vi "GetProbePlanCoordinates.vi"(8 "Use index as X coord":bool=TRUE, 9 "Probe Card Channels":i32=1) -> (0 "file path":string, 2 "OK?":bool, 3 "Array":T1(array[cluster]))   [LabVIEW 2018] (continued)
662\tX=42477.91\ty=10510.80 \nLabel=Strip\t663\tX=42126.23\ty=10577.37 \nLabel=Strip\t664\tX=42473.81\ty=10675.69 \nLabel=Strip\t665\tX=42122.11\ty=10742.12 \nLabel=Strip\t666\tX=42469.65\ty=10840.57 \nLabel=Strip\t667\tX=42117.92\ty=10906.87 \nLabel=Strip\t668\tX=42465.43\ty=11005.45 \nLabel=Strip\t669\tX=42113.68\ty=11071.62 \nLabel=Strip\t670\tX=42461.15\ty=11170.33 \nLabel=Strip\t671\tX=42109.37\ty=11236.36 \nLabel=Strip\t672\tX=42456.80\ty=11335.21 \nLabel=Strip\t673\tX=42104.99\ty=11401.11 \nLabel=Strip\t674\tX=42452.39\ty=11500.10 \nLabel=Strip\t675\tX=42100.55\ty=11565.85 \nLabel=Strip\t676\tX=42447.91\ty=11664.98 \nLabel=Strip\t677\tX=42096.05\ty=11730.60 \nLabel=Strip\t678\tX=42443.37\ty=11829.86 \nLabel=Strip\t679\tX=42091.49\ty=11895.34 \nLabel=Strip\t680\tX=42438.77\ty=11994.74 \nLabel=Strip\t681\tX=42086.86\ty=12060.09 \nLabel=Strip\t682\tX=42434.10\ty=12159.62 \nLabel=Strip\t683\tX=42082.16\ty=12224.83 \nLabel=Strip\t684\tX=42429.37\ty=12324.50 \nLabel=Strip\t685\tX=42077.41\ty=12389.58 \nLabel=Strip\t686\tX=42424.57\ty=12489.37 \nLabel=Strip\t687\tX=42072.59\ty=12554.32 \nLabel=Strip\t688\tX=42419.71\ty=12654.25 \nLabel=Strip\t689\tX=42067.70\ty=12719.06 \nLabel=Strip\t690\tX=42414.79\ty=12819.13 \nLabel=Strip\t691\tX=42062.75\ty=12883.80 \nLabel=Strip\t692\tX=42409.80\ty=12984.01 \nLabel=Strip\t693\tX=42057.74\ty=13048.55 \nLabel=Strip\t694\tX=42404.75\ty=13148.88 \nLabel=Strip\t695\tX=42052.67\ty=13213.29 \nLabel=Strip\t696\tX=42399.64\ty=13313.76 \nLabel=Strip\t697\tX=42047.53\ty=13378.03 \nLabel=Strip\t698\tX=42394.46\ty=13478.63 \nLabel=Strip\t699\tX=42042.33\ty=13542.77 \nLabel=Strip\t700\tX=42389.22\ty=13643.51 \nLabel=Strip\t701\tX=42037.06\ty=13707.50 \nLabel=Strip\t702\tX=42383.91\ty=13808.38 \nLabel=Strip\t703\tX=42031.73\ty=13872.24 \nLabel=Strip\t704\tX=42378.54\ty=13973.25 \nLabel=Strip\t705\tX=42026.34\ty=14036.98 \nLabel=Strip\t706\tX=42373.11\ty=14138.12 \nLabel=Strip\t707\tX=42020.88\ty=14201.72 \nLabel=Strip\t708\tX=42367.61\ty=14302.99 \nLabel=Strip\t709\tX=42015.36\ty=14366.45 \nLabel=Strip\t710\tX=42362.05\ty=14467.86 \nLabel=Strip\t711\tX=42009.77\ty=14531.19 \nLabel=Strip\t712\tX=42356.43\ty=14632.73 \nLabel=Strip\t713\tX=42004.12\ty=14695.92 \nLabel=Strip\t714\tX=42350.74\ty=14797.60 \nLabel=Strip\t715\tX=41998.41\ty=14860.65 \nLabel=Strip\t716\tX=42344.99\ty=14962.47 \nLabel=Strip\t717\tX=41992.63\ty=15025.38 \nLabel=Strip\t718\tX=42339.17\ty=15127.33 \nLabel=Strip\t719\tX=41986.79\ty=15190.12 \nLabel=Strip\t720\tX=42333.29\ty=15292.20 \nLabel=Strip\t721\tX=41980.89\ty=15354.85 \nLabel=Strip\t722\tX=42327.35\ty=15457.06 \nLabel=Strip\t723\tX=41974.92\ty=15519.57 \nLabel=Strip\t724\tX=42321.34\ty=15621.93 \nLabel=Strip\t725\tX=41968.89\ty=15684.30 \nLabel=Strip\t726\tX=42315.27\ty=15786.79 \nLabel=Strip\t727\tX=41962.80\ty=15849.03 \nLabel=Strip\t728\tX=42309.14\ty=15951.65 \nLabel=Strip\t729\tX=41956.64\ty=16013.76 \nLabel=Strip\t730\tX=42302.94\ty=16116.51 \nLabel=Strip\t731\tX=41950.42\ty=16178.48 \nLabel=Strip\t732\tX=42296.68\ty=16281.37 \nLabel=Strip\t733\tX=41944.08\ty=16344.03 \nLabel=Strip\t734\tX=42290.35\ty=16446.23 \nLabel=Strip\t735\tX=41937.78\ty=16507.93 \nLabel=Strip\t736\tX=42283.96\ty=16611.09 \nLabel=Strip\t737\tX=41931.37\ty=16672.65 \nLabel=Strip\t738\tX=42277.51\ty=16775.94 \nLabel=Strip\t739\tX=41924.89\ty=16837.37 \nLabel=Strip\t740\tX=42270.99\ty=16940.80 \nLabel=Strip\t741\tX=41918.35\ty=17002.09 \nLabel=Strip\t742\tX=42264.41\ty=17105.65 \nLabel=Strip\t743\tX=41911.74\ty=17166.81 \nLabel=Strip\t744\tX=42257.77\ty=17270.50 \nLabel=Strip\t745\tX=41905.08\ty=17331.52 \nLabel=Strip\t746\tX=42251.06\ty=17435.35 \nLabel=Strip\t747\tX=41898.34\ty=17496.24 \nLabel=Strip\t748\tX=42244.29\ty=17600.20 \nLabel=Strip\t749\tX=41891.55\ty=17660.95 \nLabel=Strip\t750\tX=42237.45\ty=17765.05 \nLabel=Strip\t751\tX=41884.69\ty=17825.66 \nLabel=Strip\t752\tX=42230.55\ty=17929.90 \nLabel=Strip\t753\tX=41877.77\ty=17990.37 \nLabel=Strip\t754\tX=42223.59\ty=18094.74 \nLabel=Strip\t755\tX=41870.78\ty=18155.08 \nLabel=Strip\t756\tX=42216.56\ty=18259.59 \nLabel=Strip\t757\tX=41863.73\ty=18319.79 \nLabel=Strip\t758\tX=42209.47\ty=18424.43 \nLabel=Strip\t759\tX=41856.61\ty=18484.50 \nLabel=Strip\t760\tX=42202.31\ty=18589.27 \nLabel=Strip\t761\tX=41849.43\ty=18649.21 \nLabel=Strip\t762\tX=42195.09\ty=18754.11 \nLabel=Strip\t763\tX=41842.19\ty=18813.91 \nLabel=Strip\t764\tX=42187.81\ty=18918.95 \nLabel=Strip\t765\tX=41834.89\ty=18978.61 \nLabel=Strip\t766\tX=42180.47\ty=19083.79 \nLabel=Strip\t767\tX=41827.52\ty=19143.31 \nLabel=Strip\t768\tX=42173.06\ty=19248.62 \nLabel=Strip\t769\tX=41820.08\ty=19308.01 \nLabel=Strip\t770\tX=42165.58\ty=19413.45 \nLabel=Strip\t771\tX=41812.59\ty=19472.71 \nLabel=Strip\t772\tX=42158.04\ty=19578.29 \nLabel=Strip\t773\tX=41805.03\ty=19637.41 \nLabel=Strip\t774\tX=42150.44\ty=19743.12 \nLabel=Strip\t775\tX=41797.40\ty=19802.10 \nLabel=Strip\t776\tX=42142.78\ty=19907.95 \nLabel=Strip\t777\tX=41789.71\ty=19966.79 \nLabel=Strip\t778\tX=42135.05\ty=20072.77 \nLabel=Strip\t779\tX=41781.96\ty=20131.49 \nLabel=Strip\t780\tX=42127.26\ty=20237.60 \nLabel=Strip\t781\tX=41774.15\ty=20296.18 \nLabel=Strip\t782\tX=42119.40\ty=20402.42 \nLabel=Strip\t783\tX=41766.27\ty=20460.86 \nLabel=Strip\t784\tX=42111.48\ty=20567.24 \nLabel=Strip\t785\tX=41758.33\ty=20625.55 \nLabel=Strip\t786\tX=42103.49\ty=20732.06 \nLabel=Strip\t787\tX=41750.32\ty=20790.23 \nLabel=Strip\t788\tX=42095.45\ty=20896.88 \nLabel=Strip\t789\tX=41742.25\ty=20954.92 \nLabel=Strip\t790\tX=42087.33\ty=21061.70 \nLabel=Strip\t791\tX=41734.11\ty=21119.60 \nLabel=Strip\t792\tX=42079.16\ty=21226.51 \nLabel=Strip\t793\tX=41725.92\ty=21284.28 \nLabel=Strip\t794\tX=42070.92\ty=21391.33 \nLabel=Strip\t795\tX=41717.65\ty=21448.95 \nLabel=Strip\t796\tX=42062.62\ty=21556.14 \nLabel=Strip\t797\tX=41709.33\ty=21613.63 \nLabel=Strip\t798\tX=42054.25\ty=21720.95 \nLabel=Strip\t799\tX=41700.94\ty=21778.30 \nLabel=Strip\t800\tX=42045.82\ty=21885.75 \nLabel=Strip\t801\tX=41692.49\ty=21942.97 \nLabel=Strip\t802\tX=42037.32\ty=22050.56 \nLabel=Strip\t803\tX=41683.97\ty=22107.64 \nLabel=Strip\t804\tX=42028.77\ty=22215.36 \nLabel=Strip\t805\tX=41675.39\ty=22272.31 \nLabel=Strip\t806\tX=42020.14\ty=22380.16 \nLabel=Strip\t807\tX=41666.74\ty=22436.97 \nLabel=Strip\t808\tX=42011.46\ty=22544.96 \nLabel=Strip\t809\tX=41658.04\ty=22601.64 \nLabel=Strip\t810\tX=42002.71\ty=22709.76 \nLabel=Strip\t811\tX=41649.26\ty=22766.30 \nLabel=Strip\t812\tX=41993.89\ty=22874.55 \nLabel=Strip\t813\tX=41640.43\ty=22930.96 \nLabel=Strip\t814\tX=41985.02\ty=23039.34 \nLabel=Strip\t815\tX=41631.53\ty=23095.61 \nLabel=Strip\t816\tX=41976.07\ty=23204.14 \nLabel=Strip\t817\tX=41622.57\ty=23260.27 \nLabel=Strip\t818\tX=41967.07\ty=23368.92 \nLabel=Strip\t819\tX=41613.54\ty=23424.92 \nLabel=Strip\t820\tX=41958.00\ty=23533.71 \nLabel=Strip\t821\tX=41604.45\ty=23589.57 \nLabel=Strip\t822\tX=41948.87\ty=23698.49 \nLabel=Strip\t823\tX=41595.30\ty=23754.22 \nLabel=Strip\t824\tX=41939.67\ty=23863.28 \nLabel=Strip\t825\tX=41586.08\ty=23918.87 \nLabel=Strip\t826\tX=41930.41\ty=24028.06 \nLabel=Strip\t827\tX=41576.79\ty=24083.51 \nLabel=Strip\t828\tX=41921.09\ty=24192.83 \nLabel=Strip\t829\tX=41567.45\ty=24248.15 \nLabel=Strip\t830\tX=41911.70\ty=24357.61 \nLabel=Strip\t831\tX=41558.04\ty=24412.79 \nLabel=Strip\t832\tX=41902.25\ty=24522.38 \nLabel=Strip\t833\tX=41548.57\ty=24577.43 \nLabel=Strip\t834\tX=41892.73\ty=24687.15 \nLabel=Strip\t835\tX=41539.03\ty=24742.06 \nLabel=Strip\t836\tX=41883.15\ty=24851.92 \nLabel=Strip\t837\tX=41529.43\ty=24906.69 \nLabel=Strip\t838\tX=41873.51\ty=25016.68 \nLabel=Strip\t839\tX=41519.77\ty=25071.32 \nLabel=Strip\t840\tX=41863.80\ty=25181.45 \nLabel=Strip\t841\tX=41510.04\ty=25235.95 \nLabel=Strip\t842\tX=41854.03\ty=25346.21 \nLabel=Strip\t843\tX=41500.25\ty=25400.57 \nLabel=Strip\t844\tX=41844.20\ty=25510.96 \nLabel=Strip\t845\tX=41490.39\ty=25565.20 \nLabel=Strip\t846\tX=41834.30\ty=25675.72 \nLabel=Strip\t847\tX=41480.47\ty=25729.82 \nLabel=Strip\t848\tX=41824.34\ty=25840.47 \nLabel=Strip\t849\tX=41470.49\ty=25894.43 \nLabel=Strip\t850\tX=41814.31\ty=26005.22 \nLabel=Strip\t851\tX=41460.44\ty=26059.05 \nLabel=Strip\t852\tX=41804.22\ty=26169.97 \nLabel=Strip\t853\tX=41450.33\ty=26223.66 \nLabel=Strip\t854\tX=41794.07\ty=26334.72 \nLabel=Strip\t855\tX=41440.16\ty=26388.27 \nLabel=Strip\t856\tX=41783.85\ty=26499.46 \nLabel=Strip\t857\tX=41429.92\ty=26552.87 \nLabel=Strip\t858\tX=41773.57\ty=26664.20 \nLabel=Strip\t859\tX=41419.62\ty=26717.48 \nLabel=Strip\t860\tX=41763.23\ty=26828.94 \nLabel=Strip\t861\tX=41409.25\ty=26882.08 \nLabel=Strip\t862\tX=41752.82\ty=26993.67 \nLabel=Strip\t863\tX=41398.82\ty=27046.68 \nLabel=Strip\t864\tX=41742.35\ty=27158.40 \nLabel=Strip\t865\tX=41388.33\ty=27211.27 \nLabel=Strip\t866\tX=41731.81\ty=27323.13 \nLabel=Strip\t867\tX=41377.78\ty=27375.87 \nLabel=Strip\t868\tX=41721.21\ty=27487.86 \nLabel=Strip\t869\tX=41367.16\ty=27540.46 \nLabel=Strip\t870\tX=41710.55\ty=27652.58 \nLabel=Strip\t871\tX=41356.47\ty=27705.04 \nLabel=Strip\t872\tX=41699.82\ty=27817.30 \nLabel=Strip\t873\tX=41345.72\ty=27869.63 \nLabel=Strip\t874\tX=41689.03\ty=27982.02 \nLabel=Strip\t875\tX=41334.91\ty=28034.21 \nLabel=Strip\t876\tX=41678.17\ty=28146.73 \nLabel=Strip\t877\tX=41324.04\ty=28198.79 \nLabel=Strip\t878\tX=41667.25\ty=28311.45 \nLabel=Strip\t879\tX=41313.10\ty=28363.36 \nLabel=Strip\t880\tX=41656.27\ty=28476.15 \nLabel=Strip\t881\tX=41302.09\ty=28527.94 \nLabel=Strip\t882\tX=41645.22\ty=28640.86 \nLabel=Strip\t883\tX=41291.03\ty=28692.51 \nLabel=Strip\t884\tX=41634.11\ty=28805.61 \nLabel=Strip\t885\tX=41279.90\ty=28857.07 \nLabel=Strip\t886\tX=41622.94\ty=28970.26 \nLabel=Strip\t887\tX=41268.70\ty=29021.64 \nLabel=Strip\t888\tX=41611.70\ty=29134.96 \nLabel=Strip\t889\tX=41257.45\ty=29186.20 \nLabel=Strip\t890\tX=41600.40\ty=29299.66 \nLabel=Strip\t891\tX=41246.12\ty=29350.76 \nLabel=Strip\t892\tX=41589.04\ty=29464.35 \nLabel=Strip\t893\tX=41234.74\ty=29515.31 \nLabel=Strip\t894\tX=41577.59\ty=29629.21 \nLabel=Strip\t895\tX=41223.29\ty=29679.86 \nLabel=Strip\t896\tX=41566.11\ty=29793.72 \nLabel=Strip\t897\tX=41211.78\ty=29844.41 \nLabel=Strip\t898\tX=41554.56\ty=29958.40 \nLabel=Strip\t899\tX=41200.20\ty=30008.96 \nLabel=Strip\t900\tX=41542.94\ty=30123.08 \nLabel=Strip\t901\tX=41188.56\ty=30173.50 \nLabel=Strip\t902\tX=41531.25\ty=30287.75 \nLabel=Strip\t903\tX=41176.86\ty=30338.04 \nLabel=Strip\t904\tX=41519.50\ty=30452.43 \nLabel=Strip\t905\tX=41165.09\ty=30502.57 \nLabel=Strip\t906\tX=41507.69\ty=30617.09 \nLabel=Strip\t907\tX=41153.26\ty=30667.11 \nLabel=Strip\t908\tX=41495.82\ty=30781.76 \nLabel=Strip\t909\tX=41141.36\ty=30831.63 \nLabel=Strip\t910\tX=41483.88\ty=30946.42 \nLabel=Strip\t911\tX=41129.40\ty=30996.16 \nLabel=Strip\t912\tX=41471.87\ty=31111.08 \nLabel=Strip\t913\tX=41117.38\ty=31160.68 \nLabel=Strip\t914\tX=41459.80\ty=31275.73 \nLabel=Strip\t915\tX=41105.29\ty=31325.20 \nLabel=Strip\t916\tX=41447.67\ty=31440.39 \nLabel=Strip\t917\tX=41093.14\ty=31489.72 \nLabel=Strip\t918\tX=41435.48\ty=31605.04 \nLabel=Strip\t919\tX=41080.93\ty=31654.23 \nLabel=Strip\t920\tX=41423.22\ty=31769.68 \nLabel=Strip\t921\tX=41068.65\ty=31818.74 \nLabel=Strip\t922\tX=41410.90\ty=31934.32 \nLabel=Strip\t923\tX=41056.31\ty=31983.24 \nLabel=Strip\t924\tX=41398.51\ty=32098.96 \nLabel=Strip\t925\tX=41043.90\ty=32147.75 \nLabel=Strip\t926\tX=41386.06\ty=32263.59 \nLabel=Strip\t927\tX=41031.44\ty=32312.24 \nLabel=Strip\t928\tX=41373.55\ty=32428.23 \nLabel=Strip\t929\tX=41018.90\ty=32476.74 \nLabel=Strip\t930\tX=41360.97\ty=32592.85 \nLabel=Strip\t931\tX=41006.31\ty=32641.23 \nLabel=Strip\t932\tX=41348.33\ty=32757.48 \nLabel=Strip\t933\tX=40993.65\ty=32805.72 \nLabel=Strip\t934\tX=41335.62\ty=32922.10 \nLabel=Strip\t935\tX=40980.92\ty=32970.20 \nLabel=Strip\t936\tX=41322.86\ty=33086.71 \nLabel=Strip\t937\tX=40968.14\ty=33134.68 \nLabel=Strip\t938\tX=41310.02\ty=33251.33 \nLabel=Strip\t939\tX=40955.28\ty=33299.16 \nLabel=Strip\t940\tX=41297.13\ty=33415.94 \nLabel=Strip\t941\tX=40942.37\ty=33463.63 \nLabel=Strip\t942\tX=41284.17\ty=33580.54 \nLabel=Strip\t943\tX=40929.39\ty=33628.10 \nLabel=Strip\t944\tX=41271.14\ty=33745.14 \nLabel=Strip\t945\tX=40916.35\ty=33792.57 \nLabel=Strip\t946\tX=41258.05\ty=33909.74 \nLabel=Strip\t947\tX=40903.24\ty=33957.03 \nLabel=Strip\t948\tX=41244.90\ty=34074.34 \nLabel=Strip\t949\tX=40890.07\ty=34121.49 \nLabel=Strip\t950\tX=41231.69\ty=34238.93 \nLabel=Strip\t951\tX=40876.84\ty=34285.94 \nLabel=Strip\t952\tX=41218.41\ty=34403.52 \nLabel=Strip\t953\tX=40863.54\ty=34450.39 \nLabel=Strip\t954\tX=41205.06\ty=34568.10 \nLabel=Strip\t955\tX=40850.18\ty=34614.84 \nLabel=Strip\t956\tX=41191.66\ty=34732.68 \nLabel=Strip\t957\tX=40836.75\ty=34779.28 \nLabel=Strip\t958\tX=41178.19\ty=34897.25 \nLabel=Strip\t959\tX=40823.27\ty=34943.72 \nLabel=Strip\t960\tX=41164.65\ty=35061.82 \nLabel=Strip\t961\tX=40809.71\ty=35108.15 \nLabel=Strip\t962\tX=41151.05\ty=35226.39 \nLabel=Strip\t963\tX=40796.10\ty=35272.59 \nLabel=Strip\t964\tX=41137.39\ty=35390.95 \nLabel=Strip\t965\tX=40782.42\ty=35437.01 \nLabel=Strip\t966\tX=41123.67\ty=35555.51 \nLabel=Strip\t967\tX=40768.67\ty=35601.43 \nLabel=Strip\t968\tX=41109.88\ty=35720.07 \nLabel=Strip\t969\tX=40754.87\ty=35765.85 \nLabel=Strip\t970\tX=41096.02\ty=35884.62 \nLabel=Strip\t971\tX=40741.00\ty=35930.27 \nLabel=Strip\t972\tX=41082.11\ty=36049.17 \nLabel=Strip\t973\tX=40727.06\ty=36094.68 \nLabel=Strip\t974\tX=41068.13\ty=36213.71 \nLabel=Strip\t975\tX=40713.06\ty=36259.09 \nLabel=Strip\t976\tX=41054.08\ty=36378.25 \nLabel=Strip\t977\tX=40699.00\ty=36423.49 \nLabel=Strip\t978\tX=41039.97\ty=36542.78 \nLabel=Strip\t979\tX=40684.87\ty=36587.89 \nLabel=Strip\t980\tX=41025.80\ty=36707.31 \nLabel=Strip\t981\tX=40670.68\ty=36752.28 \nLabel=Strip\t982\tX=41011.57\ty=36871.84 \nLabel=Strip\t983\tX=40656.43\ty=36916.67 \nLabel=Strip\t984\tX=40997.27\ty=37036.36 \nLabel=Strip\t985\tX=40642.11\ty=37081.06 \nLabel=Strip\t986\tX=40982.90\ty=37200.88 \nLabel=Strip\t987\tX=40627.73\ty=37245.44 \nLabel=Strip\t988\tX=40968.48\ty=37365.39 \nLabel=Strip\t989\tX=40613.29\ty=37409.82 \nLabel=Strip\t990\tX=40953.98\ty=37529.90 \nLabel=Strip\t991\tX=40598.78\ty=37574.19 \nLabel=Strip\t992\tX=40939.43\ty=37694.41 \nLabel=Strip\t993\tX=40584.21\ty=37738.56 \nLabel=Strip\t994\tX=40924.81\ty=37858.91 \nLabel=Strip\t995\tX=40569.57\ty=37902.92 \nLabel=Strip\t996\tX=40910.13\ty=38023.41 \nLabel=Strip\t997\tX=40554.87\ty=38067.28 \nLabel=Strip\t998\tX=40895.38\ty=38187.90 \nLabel=Strip\t999\tX=40540.11\ty=38231.64 \nLabel=Strip\t1000\tX=40880.57\ty=38352.39 \nLabel=Strip\t1001\tX=40525.28\ty=38395.99 \nLabel=Strip\t1002\tX=40865.70\ty=38516.87 \nLabel=Strip\t1003\tX=40510.39\ty=38560.33 \nLabel=Strip\t1004\tX=40850.76\ty=38681.35 \nLabel=Strip\t1005\tX=40495.44\ty=38724.68 \nLabel=Strip\t1006\tX=40835.76\ty=38845.82 \nLabel=Strip\t1007\tX=40480.42\ty=38889.01 \nLabel=Strip\t1008\tX=40820.69\ty=39010.29 \nLabel=Strip\t1009\tX=40465.34\ty=39053.35 \nLabel=Strip\t1010\tX=40805.57\ty=39174.76 \nLabel=Strip\t1011\tX=40450.19\ty=39217.67 \nLabel=Strip\t1012\tX=40790.37\ty=39339.22 \nLabel=Strip\t1013\tX=40434.98\ty=39382.00 \nLabel=Strip\t1014\tX=40775.12\ty=39503.67 \nLabel=Strip\t1015\tX=40419.71\ty=39546.32 \nLabel=Strip\t1016\tX=40759.80\ty=39668.12 \nLabel=Strip\t1017\tX=40404.37\ty=39710.63 \nLabel=Strip\t1018\tX=40744.41\ty=39832.57 \nLabel=Strip\t1019\tX=40388.97\ty=39874.94 \nLabel=Strip\t1020\tX=40728.97\ty=39997.01 \nLabel=Strip\t1021\tX=40373.51\ty=40039.25 \nLabel=Strip\t1022\tX=40713.45\ty=40161.45 \nLabel=Strip\t1023\tX=40357.98\ty=40203.55 \nLabel=Strip\t1024\tX=40697.88\ty=40325.88 \nLabel=Strip\t1025\tX=40342.39\ty=40367.84 \nLabel=Strip\t1026\tX=40682.24\ty=40490.31 \nRegion=Segment\t1T\nLabel=Strip\t1\tX=41752.70\ty=-43974.75 \nLabel=Strip\t2\tX=42109.05\ty=-43930.54 \nLabel=Strip\t3\tX=41767.75\ty=-43828.77 \nLabel=Strip\t4\tX=42124.08\ty=-43784.43 \nLabel=Strip\t5\tX=41782.75\ty=-43682.78 \nLabel=Strip\t6\tX=42139.06\ty=-43638.32 \nLabel=Strip\t7\tX=41797.69\ty=-43536.79 \nLabel=Strip\t8\tX=42153.99\ty=-43492.20 \nLabel=Strip\t9\tX=41812.59\ty=-43390.79 \nLabel=Strip\t10\tX=42168.88\ty=-43346.08 \nLabel=Strip\t11\tX=41827.44\ty=-43244.78 \nLabel=Strip\t12\tX=42183.71\ty=-43199.95 \nLabel=Strip\t13\tX=41842.24\ty=-43098.77 \nLabel=Strip\t14\tX=42198.49\ty=-43053.82 \nLabel=Strip\t15\tX=41856.99\ty=-42952.75 \nLabel=Strip\t16\tX=42213.22\ty=-42907.68 \nLabel=Strip\t17\tX=41871.68\ty=-42806.73 \nLabel=Strip\t18\tX=42227.91\ty=-42761.53 \nLabel=Strip\t19\tX=41886.33\ty=-42660.70 \nLabel=Strip\t20\tX=42242.54\ty=-42615.38 \nLabel=Strip\t21\tX=41900.93\ty=-42514.66 \nLabel=Strip\t22\tX=42257.12\ty=-42469.22 \nLabel=Strip\t23\tX=41915.48\ty=-42368.62 \nLabel=Strip\t24\tX=42271.65\ty=-42323.05 \nLabel=Strip\t25\tX=41929.98\ty=-42222.57 \nLabel=Strip\t26\tX=42286.14\ty=-42176.88 \nLabel=Strip\t27\tX=41944.42\ty=-42076.51 \nLabel=Strip\t28\tX=42300.57\ty=-42030.70 \nLabel=Strip\t29\tX=41958.82\ty=-41930.45 \nLabel=Strip\t30\tX=42314.95\ty=-41884.52 \nLabel=Strip\t31\tX=41973.17\ty=-41784.39 \nLabel=Strip\t32\tX=42329.28\ty=-41738.33 \nLabel=Strip\t33\tX=41987.47\ty=-41638.32 \nLabel=Strip\t34\tX=42343.57\ty=-41592.14 \nLabel=Strip\t35\tX=42001.72\ty=-41492.24 \nLabel=Strip\t36\tX=42357.80\ty=-41445.93 \nLabel=Strip\t37\tX=42015.91\ty=-41346.15 \nLabel=Strip\t38\tX=42371.98\ty=-41299.73 \nLabel=Strip\t39\tX=42030.06\ty=-41200.06 \nLabel=Strip\t40\tX=42386.11\ty=-41153.51 \nLabel=Strip\t41\tX=42044.16\ty=-41053.97 \nLabel=Strip\t42\tX=42400.20\ty=-41007.30 \nLabel=Strip\t43\tX=42058.21\ty=-40907.86 \nLabel=Strip\t44\tX=42414.23\ty=-40861.07 \nLabel=Strip\t45\tX=42072.21\ty=-40761.76 \nLabel=Strip\t46\tX=42428.21\ty=-40714.84 \nLabel=Strip\t47\tX=42086.16\ty=-40615.64 \nLabel=Strip\t48\tX=42442.14\ty=-40568.60 \nLabel=Strip\t49\tX=42100.05\ty=-40469.52 \nLabel=Strip\t50\tX=42456.03\ty=-40422.36 \nLabel=Strip\t51\tX=42113.90\ty=-40323.40 \nLabel=Strip\t52\tX=42469.86\ty=-40276.11 \nLabel=Strip\t53\tX=42127.70\ty=-40177.27 \nLabel=Strip\t54\tX=42483.64\ty=-40129.86 \nLabel=Strip\t55\tX=42141.45\ty=-40031.13 \nLabel=Strip\t56\tX=42497.37\ty=-39983.60 \nLabel=Strip\t57\tX=42155.15\ty=-39884.99 \nLabel=Strip\t58\tX=42511.05\ty=-39837.34 \nLabel=Strip\t59\tX=42168.80\ty=-39738.84 \nLabel=Strip\t60\tX=42524.69\ty=-39691.07 \nLabel=Strip\t61\tX=42182.39\ty=-39592.69 \nLabel=Strip\t62\tX=42538.27\ty=-39544.79 \nLabel=Strip\t63\tX=42195.94\ty=-39446.53 \nLabel=Strip\t64\tX=42551.80\ty=-39398.51 \nLabel=Strip\t65\tX=42209.44\ty=-39300.36 \nLabel=Strip\t66\tX=42565.28\ty=-39252.22 \nLabel=Strip\t67\tX=42222.89\ty=-39154.19 \nLabel=Strip\t68\tX=42578.71\ty=-39105.93 \nLabel=Strip\t69\tX=42236.29\ty=-39008.02 \nLabel=Strip\t70\tX=42592.09\ty=-38959.63 \nLabel=Strip\t71\tX=42249.64\ty=-38861.84 \nLabel=Strip\t72\tX=42605.43\ty=-38813.32 \nLabel=Strip\t73\tX=42262.93\ty=-38715.65 \nLabel=Strip\t74\tX=42618.71\ty=-38667.01 \nLabel=Strip\t75\tX=42276.18\ty=-38569.45 \nLabel=Strip\t76\tX=42631.94\ty=-38520.70 \nLabel=Strip\t77\tX=42289.38\ty=-38423.26 \nLabel=Strip\t78\tX=42645.12\ty=-38374.38 \nLabel=Strip\t79\tX=42302.53\ty=-38277.05 \nLabel=Strip\t80\tX=42658.25\ty=-38228.05 \nLabel=Strip\t81\tX=42315.63\ty=-38130.84 \nLabel=Strip\t82\tX=42671.33\ty=-38081.72 \nLabel=Strip\t83\tX=42328.67\ty=-37984.63 \nLabel=Strip\t84\tX=42684.36\ty=-37935.38 \nLabel=Strip\t85\tX=42341.67\ty=-37838.41 \nLabel=Strip\t86\tX=42697.35\ty=-37789.04 \nLabel=Strip\t87\tX=42354.62\ty=-37692.18 \nLabel=Strip\t88\tX=42710.28\ty=-37642.69 \nLabel=Strip\t89\tX=42367.52\ty=-37545.95 \nLabel=Strip\t90\tX=42723.16\ty=-37496.33 \nLabel=Strip\t91\tX=42380.37\ty=-37399.71 \nLabel=Strip\t92\tX=42735.99\ty=-37349.97 \nLabel=Strip\t93\tX=42393.16\ty=-37253.47 \nLabel=Strip\t94\tX=42748.77\ty=-37203.61 \nLabel=Strip\t95\tX=42405.91\ty=-37107.22 \nLabel=Strip\t96\tX=42761.50\ty=-37057.24 \nLabel=Strip\t97\tX=42418.61\ty=-36960.97 \nLabel=Strip\t98\tX=42774.18\ty=-36910.86 \nLabel=Strip\t99\tX=42431.26\ty=-36814.71 \nLabel=Strip\t100\tX=42786.81\ty=-36764.48 \nLabel=Strip\t101\tX=42443.85\ty=-36668.44 \nLabel=Strip\t102\tX=42799.39\ty=-36618.09 \nLabel=Strip\t103\tX=42456.40\ty=-36522.18 \nLabel=Strip\t104\tX=42811.92\ty=-36471.70 \nLabel=Strip\t105\tX=42468.90\ty=-36375.90 \nLabel=Strip\t106\tX=42824.40\ty=-36325.30 \nLabel=Strip\t107\tX=42481.35\ty=-36229.62 \nLabel=Strip\t108\tX=42836.83\ty=-36178.90 \nLabel=Strip\t109\tX=42493.74\ty=-36083.34 \nLabel=Strip\t110\tX=42849.21\ty=-36032.49 \nLabel=Strip\t111\tX=42506.09\ty=-35937.04 \nLabel=Strip\t112\tX=42861.54\ty=-35886.08 \nLabel=Strip\t113\tX=42518.39\ty=-35790.75 \nLabel=Strip\t114\tX=42873.82\ty=-35739.66 \nLabel=Strip\t115\tX=42530.64\ty=-35644.45 \nLabel=Strip\t116\tX=42886.05\ty=-35593.24 \nLabel=Strip\t117\tX=42542.83\ty=-35498.14 \nLabel=Strip\t118\tX=42898.23\ty=-35446.81 \nLabel=Strip\t119\tX=42554.98\ty=-35351.83 \nLabel=Strip\t120\tX=42910.36\ty=-35300.38 \nLabel=Strip\t121\tX=42567.08\ty=-35205.51 \nLabel=Strip\t122\tX=42922.44\ty=-35153.94 \nLabel=Strip\t123\tX=42579.12\ty=-35059.19 \nLabel=Strip\t124\tX=42934.47\ty=-35007.49 \nLabel=Strip\t125\tX=42591.12\ty=-34912.86 \nLabel=Strip\t126\tX=42946.45\ty=-34861.04 \nLabel=Strip\t127\tX=42603.07\ty=-34766.53 \nLabel=Strip\t128\tX=42958.38\ty=-34714.59 \nLabel=Strip\t129\tX=42614.96\ty=-34620.19 \nLabel=Strip\t130\tX=42970.26\ty=-34568.13 \nLabel=Strip\t131\tX=42626.81\ty=-34473.85 \nLabel=Strip\t132\tX=42982.09\ty=-34421.66 \nLabel=Strip\t133\tX=42638.61\ty=-34327.51 \nLabel=Strip\t134\tX=42993.86\ty=-34275.19 \nLabel=Strip\t135\tX=42650.35\ty=-34181.15 \nLabel=Strip\t136\tX=43005.59\ty=-34128.72 \nLabel=Strip\t137\tX=42662.05\ty=-34034.80 \nLabel=Strip\t138\tX=43017.27\ty=-33982.24 \nLabel=Strip\t139\tX=42673.69\ty=-33888.43 \nLabel=Strip\t140\tX=43028.90\ty=-33835.75 \nLabel=Strip\t141\tX=42685.29\ty=-33742.07 \nLabel=Strip\t142\tX=43040.48\ty=-33689.26 \nLabel=Strip\t143\tX=42696.84\ty=-33595.69 \nLabel=Strip\t144\tX=43052.00\ty=-33542.77 \nLabel=Strip\t145\tX=42708.33\ty=-33449.31 \nLabel=Strip\t146\tX=43063.48\ty=-33396.27 \nLabel=Strip\t147\tX=42719.78\ty=-33302.93 \nLabel=Strip\t148\tX=43074.91\ty=-33249.76 \nLabel=Strip\t149\tX=42731.17\ty=-33156.54 \nLabel=Strip\t150\tX=43086.29\ty=-33103.25 \nLabel=Strip\t151\tX=42742.52\ty=-33010.15 \nLabel=Strip\t152\tX=43097.61\ty=-32956.74 \nLabel=Strip\t153\tX=42753.81\ty=-32863.76 \nLabel=Strip\t154\tX=43108.89\ty=-32810.22 \nLabel=Strip\t155\tX=42765.06\ty=-32717.35 \nLabel=Strip\t156\tX=43120.12\ty=-32663.69 \nLabel=Strip\t157\tX=42776.25\ty=-32570.95 \nLabel=Strip\t158\tX=43131.29\ty=-32517.16 \nLabel=Strip\t159\tX=42787.40\ty=-32424.53 \nLabel=Strip\t160\tX=43142.42\ty=-32370.63 \nLabel=Strip\t161\tX=42798.49\ty=-32278.12 \nLabel=Strip\t162\tX=43153.50\ty=-32224.09 \nLabel=Strip\t163\tX=42809.54\ty=-32131.70 \nLabel=Strip\t164\tX=43164.52\ty=-32077.55 \nLabel=Strip\t165\tX=42820.53\ty=-31985.27 \nLabel=Strip\t166\tX=43175.50\ty=-31931.00 \nLabel=Strip\t167\tX=42831.48\ty=-31838.84 \nLabel=Strip\t168\tX=43186.42\ty=-31784.44 \nLabel=Strip\t169\tX=42842.37\ty=-31692.40 \nLabel=Strip\t170\tX=43197.30\ty=-31637.89 \nLabel=Strip\t171\tX=42853.21\ty=-31545.96 \nLabel=Strip\t172\tX=43208.12\ty=-31491.32 \nLabel=Strip\t173\tX=42864.01\ty=-31399.52 \nLabel=Strip\t174\tX=43218.90\ty=-31344.75 \nLabel=Strip\t175\tX=42874.75\ty=-31253.07 \nLabel=Strip\t176\tX=43229.62\ty=-31198.18 \nLabel=Strip\t177\tX=42885.45\ty=-31106.61 \nLabel=Strip\t178\tX=43240.30\ty=-31051.60 \nLabel=Strip\t179\tX=42896.09\ty=-30960.15 \nLabel=Strip\t180\tX=43250.92\ty=-30905.02 \nLabel=Strip\t181\tX=42906.68\ty=-30813.69 \nLabel=Strip\t182\tX=43261.50\ty=-30758.44 \nLabel=Strip\t183\tX=42917.22\ty=-30667.22 \nLabel=Strip\t184\tX=43272.02\ty=-30611.84 \nLabel=Strip\t185\tX=42927.72\ty=-30520.74 \nLabel=Strip\t186\tX=43282.50\ty=-30465.25 \nLabel=Strip\t187\tX=42938.16\ty=-30374.27 \nLabel=Strip\t188\tX=43292.92\ty=-30318.65 \nLabel=Strip\t189\tX=42948.55\ty=-30227.78 \nLabel=Strip\t190\tX=43303.29\ty=-30172.04 \nLabel=Strip\t191\tX=42958.90\ty=-30081.30 \nLabel=Strip\t192\tX=43313.62\ty=-30025.43 \nLabel=Strip\t193\tX=42969.19\ty=-29934.80 \nLabel=Strip\t194\tX=43323.89\ty=-29878.82 \nLabel=Strip\t195\tX=42979.43\ty=-29788.31 \nLabel=Strip\t196\tX=43334.11\ty=-29732.20 \nLabel=Strip\t197\tX=42989.62\ty=-29641.81 \nLabel=Strip\t198\tX=43344.28\ty=-29585.58 \nLabel=Strip\t199\tX=42999.76\ty=-29495.30 \nLabel=Strip\t200\tX=43354.41\ty=-29438.95 \nLabel=Strip\t201\tX=43009.85\ty=-29348.79 \nLabel=Strip\t202\tX=43364.48\ty=-29292.32 \nLabel=Strip\t203\tX=43019.90\ty=-29202.28 \nLabel=Strip\t204\tX=43374.50\ty=-29145.68 \nLabel=Strip\t205\tX=43029.89\ty=-29055.76 \nLabel=Strip\t206\tX=43384.47\ty=-28999.04 \nLabel=Strip\t207\tX=43039.83\ty=-28909.23 \nLabel=Strip\t208\tX=43394.39\ty=-28852.39 \nLabel=Strip\t209\tX=43049.72\ty=-28762.71 \nLabel=Strip\t210\tX=43404.27\ty=-28705.74 \nLabel=Strip\t211\tX=43059.56\ty=-28616.17 \nLabel=Strip\t212\tX=43414.09\ty=-28559.09 \nLabel=Strip\t213\tX=43069.35\ty=-28469.64 \nLabel=Strip\t214\tX=43423.86\ty=-28412.43 \nLabel=Strip\t215\tX=43079.09\ty=-28323.10 \nLabel=Strip\t216\tX=43433.58\ty=-28265.77 \nLabel=Strip\t217\tX=43088.78\ty=-28176.55 \nLabel=Strip\t218\tX=43443.25\ty=-28119.10 \nLabel=Strip\t219\tX=43098.42\ty=-28030.00 \nLabel=Strip\t220\tX=43452.87\ty=-27972.43 \nLabel=Strip\t221\tX=43108.01\ty=-27883.45 \nLabel=Strip\t222\tX=43462.44\ty=-27825.75 \nLabel=Strip\t223\tX=43117.55\ty=-27736.89 \nLabel=Strip\t224\tX=43471.96\ty=-27679.07 \nLabel=Strip\t225\tX=43127.04\ty=-27590.33 \nLabel=Strip\t226\tX=43481.43\ty=-27532.39 \nLabel=Strip\t227\tX=43136.48\ty=-27443.76 \nLabel=Strip\t228\tX=43490.85\ty=-27385.70 \nLabel=Strip\t229\tX=43145.87\ty=-27297.19 \nLabel=Strip\t230\tX=43500.22\ty=-27239.00 \nLabel=Strip\t231\tX=43155.20\ty=-27150.61 \nLabel=Strip\t232\tX=43509.53\ty=-27092.30 \nLabel=Strip\t233\tX=43164.49\ty=-27004.03 \nLabel=Strip\t234\tX=43518.80\ty=-26945.60 \nLabel=Strip\t235\tX=43173.73\ty=-26857.45 \nLabel=Strip\t236\tX=43528.02\ty=-26798.90 \nLabel=Strip\t237\tX=43182.92\ty=-26710.86 \nLabel=Strip\t238\tX=43537.19\ty=-26652.19 \nLabel=Strip\t239\tX=43192.06\ty=-26564.27 \nLabel=Strip\t240\tX=43546.31\ty=-26505.47 \nLabel=Strip\t241\tX=43201.14\ty=-26417.67 \nLabel=Strip\t242\tX=43555.37\ty=-26358.75 \nLabel=Strip\t243\tX=43210.18\ty=-26271.07 \nLabel=Strip\t244\tX=43564.39\ty=-26212.03 \nLabel=Strip\t245\tX=43219.17\ty=-26124.47 \nLabel=Strip\t246\tX=43573.36\ty=-26065.30 \nLabel=Strip\t247\tX=43228.10\ty=-25977.86 \nLabel=Strip\t248\tX=43582.27\ty=-25918.57 \nLabel=Strip\t249\tX=43236.99\ty=-25831.24 \nLabel=Strip\t250\tX=43591.14\ty=-25771.84 \nLabel=Strip\t251\tX=43245.83\ty=-25684.63 \nLabel=Strip\t252\tX=43599.96\ty=-25625.10 \nLabel=Strip\t253\tX=43254.61\ty=-25538.01 \nLabel=Strip\t254\tX=43608.72\ty=-25478.36 \nLabel=Strip\t255\tX=43263.35\ty=-25391.38 \nLabel=Strip\t256\tX=43617.44\ty=-25331.61 \nLabel=Strip\t257\tX=43272.04\ty=-25244.75 \nLabel=Strip\t258\tX=43626.10\ty=-25184.86 \nLabel=Strip\t259\tX=43280.67\ty=-25098.12 \nLabel=Strip\t260\tX=43634.72\ty=-25038.10 \nLabel=Strip\t261\tX=43289.26\ty=-24951.48 \nLabel=Strip\t262\tX=43643.28\ty=-24891.34 \nLabel=Strip\t263\tX=43297.79\ty=-24804.84 \nLabel=Strip\t264\tX=43651.80\ty=-24744.58 \nLabel=Strip\t265\tX=43306.27\ty=-24658.20 \nLabel=Strip\t266\tX=43660.26\ty=-24597.81 \nLabel=Strip\t267\tX=43314.71\ty=-24511.55 \nLabel=Strip\t268\tX=43668.67\ty=-24451.04 \nLabel=Strip\t269\tX=43323.09\ty=-24364.89 \nLabel=Strip\t270\tX=43677.04\ty=-24304.27 \nLabel=Strip\t271\tX=43331.43\ty=-24218.24 \nLabel=Strip\t272\tX=43685.35\ty=-24157.49 \nLabel=Strip\t273\tX=43339.71\ty=-24071.58 \nLabel=Strip\t274\tX=43693.61\ty=-24010.71 \nLabel=Strip\t275\tX=43347.94\ty=-23924.91 \nLabel=Strip\t276\tX=43701.82\ty=-23863.92 \nLabel=Strip\t277\tX=43356.13\ty=-23778.24 \nLabel=Strip\t278\tX=43709.99\ty=-23717.13 \nLabel=Strip\t279\tX=43364.26\ty=-23631.57 \nLabel=Strip\t280\tX=43718.10\ty=-23570.33 \nLabel=Strip\t281\tX=43372.34\ty=-23484.90 \nLabel=Strip\t282\tX=43726.16\ty=-23423.54 \nLabel=Strip\t283\tX=43380.38\ty=-23338.22 \nLabel=Strip\t284\tX=43734.17\ty=-23276.73 \nLabel=Strip\t285\tX=43388.36\ty=-23191.53 \nLabel=Strip\t286\tX=43742.13\ty=-23129.93 \nLabel=Strip\t287\tX=43396.29\ty=-23044.84 \nLabel=Strip\t288\tX=43750.04\ty=-22983.12 \nLabel=Strip\t289\tX=43404.17\ty=-22898.15 \nLabel=Strip\t290\tX=43757.90\ty=-22836.31 \nLabel=Strip\t291\tX=43412.00\ty=-22751.46 \nLabel=Strip\t292\tX=43765.71\ty=-22689.49 \nLabel=Strip\t293\tX=43419.78\ty=-22604.76 \nLabel=Strip\t294\tX=43773.47\ty=-22542.67 \nLabel=Strip\t295\tX=43427.51\ty=-22458.06 \nLabel=Strip\t296\tX=43781.18\ty=-22395.84 \nLabel=Strip\t297\tX=43435.19\ty=-22311.35 \nLabel=Strip\t298\tX=43788.84\ty=-22249.02 \nLabel=Strip\t299\tX=43442.82\ty=-22164.64 \nLabel=Strip\t300\tX=43796.45\ty=-22102.19 \nLabel=Strip\t301\tX=43450.40\ty=-22017.93 \nLabel=Strip\t302\tX=43804.01\ty=-21955.35 \nLabel=Strip\t303\tX=43457.93\ty=-21871.21 \nLabel=Strip\t304\tX=43811.52\ty=-21808.51 \nLabel=Strip\t305\tX=43465.41\ty=-21724.49 \nLabel=Strip\t306\tX=43818.97\ty=-21661.67 \nLabel=Strip\t307\tX=43472.84\ty=-21577.77 \nLabel=Strip\t308\tX=43826.38\ty=-21514.82 \nLabel=Strip\t309\tX=43480.22\ty=-21431.04 \nLabel=Strip\t310\tX=43833.74\ty=-21367.97 \nLabel=Strip\t311\tX=43487.55\ty=-21284.31 \nLabel=Strip\t312\tX=43841.05\ty=-21221.12 \nLabel=Strip\t313\tX=43494.83\ty=-21137.58 \nLabel=Strip\t314\tX=43848.30\ty=-21074.26 \nLabel=Strip\t315\tX=43502.05\ty=-20990.84 \nLabel=Strip\t316\tX=43855.51\ty=-20927.40 \nLabel=Strip\t317\tX=43509.23\ty=-20844.10 \nLabel=Strip\t318\tX=43862.66\ty=-20780.54 \nLabel=Strip\t319\tX=43516.36\ty=-20697.35 \nLabel=Strip\t320\tX=43869.77\ty=-20633.67 \nLabel=Strip\t321\tX=43523.44\ty=-20550.60 \nLabel=Strip\t322\tX=43876.82\ty=-20486.80 \nLabel=Strip\t323\tX=43530.46\ty=-20403.85 \nLabel=Strip\t324\tX=43883.83\ty=-20339.93 \nLabel=Strip\t325\tX=43537.44\ty=-20257.09 \nLabel=Strip\t326\tX=43890.78\ty=-20193.05 \nLabel=Strip\t327\tX=43544.36\ty=-20110.34 \nLabel=Strip\t328\tX=43897.69\ty=-20046.17 \nLabel=Strip\t329\tX=43551.24\ty=-19963.57 \nLabel=Strip\t330\tX=43904.54\ty=-19899.29 \nLabel=Strip\t331\tX=43558.06\ty=-19816.81 \nLabel=Strip\t332\tX=43911.34\ty=-19752.40 \nLabel=Strip\t333\tX=43564.84\ty=-19670.04 \nLabel=Strip\t334\tX=43918.10\ty=-19605.51 \nLabel=Strip\t335\tX=43571.56\ty=-19523.27 \nLabel=Strip\t336\tX=43924.80\ty=-19458.61 \nLabel=Strip\t337\tX=43578.24\ty=-19376.49 \nLabel=Strip\t338\tX=43931.45\ty=-19311.72 \nLabel=Strip\t339\tX=43584.86\ty=-19229.71 \nLabel=Strip\t340\tX=43938.05\ty=-19164.82 \nLabel=Strip\t341\tX=43591.44\ty=-19082.93 \nLabel=Strip\t342\tX=43944.60\ty=-19017.91 \nLabel=Strip\t343\tX=43597.96\ty=-18936.14 \nLabel=Strip\t344\tX=43951.11\ty=-18871.00 \nLabel=Strip\t345\tX=43604.43\ty=-18789.35 \nLabel=Strip\t346\tX=43957.56\ty=-18724.09 \nLabel=Strip\t347\tX=43610.86\ty=-18642.56 \nLabel=Strip\t348\tX=43963.96\ty=-18577.18 \nLabel=Strip\t349\tX=43617.23\ty=-18495.77 \nLabel=Strip\t350\tX=43970.31\ty=-18430.26 \nLabel=Strip\t351\tX=43623.55\ty=-18348.97 \nLabel=Strip\t352\tX=43976.61\ty=-18283.34 \nLabel=Strip\t353\tX=43629.82\ty=-18202.17 \nLabel=Strip\t354\tX=43982.86\ty=-18136.42 \nLabel=Strip\t355\tX=43636.04\ty=-18055.36 \nLabel=Strip\t356\tX=43989.05\ty=-17989.49 \nLabel=Strip\t357\tX=43642.21\ty=-17908.55 \nLabel=Strip\t358\tX=43995.20\ty=-17842.56 \nLabel=Strip\t359\tX=43648.34\ty=-17761.74 \nLabel=Strip\t360\tX=44001.30\ty=-17695.63 \nLabel=Strip\t361\tX=43654.41\ty=-17614.93 \nLabel=Strip\t362\tX=44007.35\ty=-17548.69 \nLabel=Strip\t363\tX=43660.43\ty=-17468.11 \nLabel=Strip\t364\tX=44013.35\ty=-17401.75 \nLabel=Strip\t365\tX=43666.40\ty=-17321.29 \nLabel=Strip\t366\tX=44019.29\ty=-17254.81 \nLabel=Strip\t367\tX=43672.31\ty=-17174.46 \nLabel=Strip\t368\tX=44025.19\ty=-17107.87 \nLabel=Strip\t369\tX=43678.18\ty=-17027.64 \nLabel=Strip\t370\tX=44031.04\ty=-16960.92 \nLabel=Strip\t371\tX=43684.00\ty=-16880.81 \nLabel=Strip\t372\tX=44036.83\ty=-16813.97 \nLabel=Strip\t373\tX=43689.77\ty=-16733.98 \nLabel=Strip\t374\tX=44042.58\ty=-16667.01 \nLabel=Strip\t375\tX=43695.49\ty=-16587.14 \nLabel=Strip\t376\tX=44048.27\ty=-16520.05 \nLabel=Strip\t377\tX=43701.16\ty=-16440.30 \nLabel=Strip\t378\tX=44053.92\ty=-16373.09 \nLabel=Strip\t379\tX=43706.77\ty=-16293.46 \nLabel=Strip\t380\tX=44059.51\ty=-16226.13 \nLabel=Strip\t381\tX=43712.34\ty=-16146.61 \nLabel=Strip\t382\tX=44065.05\ty=-16079.16 \nLabel=Strip\t383\tX=43717.86\ty=-15999.77 \nLabel=Strip\t384\tX=44070.55\ty=-15932.19 \nLabel=Strip\t385\tX=43723.32\ty=-15852.92 \nLabel=Strip\t386\tX=44075.99\ty=-15785.22 \nLabel=Strip\t387\tX=43728.74\ty=-15706.06 \nLabel=Strip\t388\tX=44081.38\ty=-15638.25 \nLabel=Strip\t389\tX=43734.10\ty=-15559.21 \nLabel=Strip\t390\tX=44086.72\ty=-15491.27 \nLabel=Strip\t391\tX=43739.42\ty=-15412.35 \nLabel=Strip\t392\tX=44092.02\ty=-15344.29 \nLabel=Strip\t393\tX=43744.68\ty=-15265.48 \nLabel=Strip\t394\tX=44097.26\ty=-15197.30 \nLabel=Strip\t395\tX=43749.90\ty=-15118.62 \nLabel=Strip\t396\tX=44102.45\ty=-15050.32 \nLabel=Strip\t397\tX=43755.06\ty=-14971.75 \nLabel=Strip\t398\tX=44107.59\ty=-14903.33 \nLabel=Strip\t399\tX=43760.18\ty=-14824.88 \nLabel=Strip\t400\tX=44112.68\ty=-14756.34 \nLabel=Strip\t401\tX=43765.24\ty=-14678.01 \nLabel=Strip\t402\tX=44117.72\ty=-14609.34 \nLabel=Strip\t403\tX=43770.25\ty=-14531.13 \nLabel=Strip\t404\tX=44122.71\ty=-14462.34 \nLabel=Strip\t405\tX=43775.21\ty=-14384.25 \nLabel=Strip\t406\tX=44127.65\ty=-14315.34 \nLabel=Strip\t407\tX=43780.13\ty=-14237.37 \nLabel=Strip\t408\tX=44132.54\ty=-14168.34 \nLabel=Strip\t409\tX=43784.99\ty=-14090.49 \nLabel=Strip\t410\tX=44137.37\ty=-14021.33 \nLabel=Strip\t411\tX=43789.80\ty=-13943.60 \nLabel=Strip\t412\tX=44142.16\ty=-13874.33 \nLabel=Strip\t413\tX=43794.56\ty=-13796.71 \nLabel=Strip\t414\tX=44146.90\ty=-13727.32 \nLabel=Strip\t415\tX=43799.27\ty=-13649.82 \nLabel=Strip\t416\tX=44151.59\ty=-13580.30 \nLabel=Strip\t417\tX=43803.93\ty=-13502.92 \nLabel=Strip\t418\tX=44156.22\ty=-13433.28 \nLabel=Strip\t419\tX=43808.54\ty=-13356.03 \nLabel=Strip\t420\tX=44160.81\ty=-13286.27 \nLabel=Strip\t421\tX=43813.10\ty=-13209.13 \nLabel=Strip\t422\tX=44165.34\ty=-13139.24 \nLabel=Strip\t423\tX=43817.61\ty=-13062.22 \nLabel=Strip\t424\tX=44169.83\ty=-12992.22 \nLabel=Strip\t425\tX=43822.07\ty=-12915.32 \nLabel=Strip\t426\tX=44174.26\ty=-12845.19 \nLabel=Strip\t427\tX=43826.48\ty=-12768.41 \nLabel=Strip\t428\tX=44178.65\ty=-12698.16 \nLabel=Strip\t429\tX=43830.83\ty=-12621.50 \nLabel=Strip\t430\tX=44182.98\ty=-12551.13 \nLabel=Strip\t431\tX=43835.14\ty=-12474.59 \nLabel=Strip\t432\tX=44187.26\ty=-12404.10 \nLabel=Strip\t433\tX=43839.40\ty=-12327.67 \nLabel=Strip\t434\tX=44191.50\ty=-12257.06 \nLabel=Strip\t435\tX=43843.60\ty=-12180.75 \nLabel=Strip\t436\tX=44195.68\ty=-12110.02 \nLabel=Strip\t437\tX=43847.76\ty=-12033.83 \nLabel=Strip\t438\tX=44199.81\ty=-11962.98 \nLabel=Strip\t439\tX=43851.87\ty=-11886.91 \nLabel=Strip\t440\tX=44203.89\ty=-11815.94 \nLabel=Strip\t441\tX=43855.92\ty=-11739.98 \nLabel=Strip\t442\tX=44207.92\ty=-11668.89 \nLabel=Strip\t443\tX=43859.93\ty=-11593.06 \nLabel=Strip\t444\tX=44211.90\ty=-11521.84 \nLabel=Strip\t445\tX=43863.88\ty=-11446.13 \nLabel=Strip\t446\tX=44215.83\ty=-11374.79 \nLabel=Strip\t447\tX=43867.79\ty=-11299.19 \nLabel=Strip\t448\tX=44219.71\ty=-11227.73 \nLabel=Strip\t449\tX=43871.64\ty=-11152.26 \nLabel=Strip\t450\tX=44223.54\ty=-11080.68 \nLabel=Strip\t451\tX=43875.44\ty=-11005.32 \nLabel=Strip\t452\tX=44227.32\ty=-10933.62 \nLabel=Strip\t453\tX=43879.19\ty=-10858.38 \nLabel=Strip\t454\tX=44231.05\ty=-10786.56 \nLabel=Strip\t455\tX=43882.90\ty=-10711.44 \nLabel=Strip\t456\tX=44234.73\ty=-10638.61 \nLabel=Strip\t457\tX=43886.55\ty=-10564.03 \nLabel=Strip\t458\tX=44238.36\ty=-10491.90 \nLabel=Strip\t459\tX=43890.15\ty=-10417.32 \nLabel=Strip\t460\tX=44241.93\ty=-10345.18 \nLabel=Strip\t461\tX=43893.70\ty=-10270.60 \nLabel=Strip\t462\tX=44245.46\ty=-10198.47 \nLabel=Strip\t463\tX=43897.20\ty=-10123.88 \nLabel=Strip\t464\tX=44248.93\ty=-10051.75 \nLabel=Strip\t465\tX=43900.65\ty=-9977.16 \nLabel=Strip\t466\tX=44252.36\ty=-9905.03 \nLabel=Strip\t467\tX=43904.05\ty=-9829.74 \nLabel=Strip\t468\tX=44255.73\ty=-9757.07 \nLabel=Strip\t469\tX=43907.40\ty=-9682.78 \nLabel=Strip\t470\tX=44259.06\ty=-9609.99 \nLabel=Strip\t471\tX=43910.70\ty=-9535.82 \nLabel=Strip\t472\tX=44262.33\ty=-9462.91 \nLabel=Strip\t473\tX=43913.95\ty=-9388.86 \nLabel=Strip\t474\tX=44265.56\ty=-9315.83 \nLabel=Strip\t475\tX=43917.15\ty=-9241.90 \nLabel=Strip\t476\tX=44268.73\ty=-9168.74 \nLabel=Strip\t477\tX=43920.30\ty=-9094.93 \nLabel=Strip\t478\tX=44271.85\ty=-9021.65 \nLabel=Strip\t479\tX=43923.39\ty=-8947.96 \nLabel=Strip\t480\tX=44274.92\ty=-8874.56 \nLabel=Strip\t481\tX=43926.44\ty=-8800.99 \nLabel=Strip\t482\tX=44277.95\ty=-8727.47 \nLabel=Strip\t483\tX=43929.44\ty=-8654.02 \nLabel=Strip\t484\tX=44280.92\ty=-8580.38 \nLabel=Strip\t485\tX=43932.38\ty=-8507.05 \nLabel=Strip\t486\tX=44283.84\ty=-8433.28 \nLabel=Strip\t487\tX=43935.28\ty=-8360.07 \nLabel=Strip\t488\tX=44286.71\ty=-8286.19 \nLabel=Strip\t489\tX=43938.12\ty=-8213.09 \nLabel=Strip\t490\tX=44289.53\ty=-8139.09 \nLabel=Strip\t491\tX=43940.92\ty=-8066.11 \nLabel=Strip\t492\tX=44292.30\ty=-7991.98 \nLabel=Strip\t493\tX=43943.66\ty=-7919.13 \nLabel=Strip\t494\tX=44295.02\ty=-7844.88 \nLabel=Strip\t495\tX=43946.36\ty=-7772.15 \nLabel=Strip\t496\tX=44297.68\ty=-7697.77 \nLabel=Strip\t497\tX=43949.00\ty=-7625.16 \nLabel=Strip\t498\tX=44300.30\ty=-7550.67 \nLabel=Strip\t499\tX=43951.59\ty=-7478.17 \nLabel=Strip\t500\tX=44302.87\ty=-7403.56 \nLabel=Strip\t501\tX=43954.14\ty=-7331.18 \nLabel=Strip\t502\tX=44305.39\ty=-7256.45 \nLabel=Strip\t503\tX=43956.63\ty=-7184.19 \nLabel=Strip\t504\tX=44307.85\ty=-7109.33 \nLabel=Strip\t505\tX=43959.07\ty=-7037.19 \nLabel=Strip\t506\tX=44310.27\ty=-6962.22 \nLabel=Strip\t507\tX=43961.46\ty=-6890.20 \nLabel=Strip\t508\tX=44312.63\ty=-6815.10 \nLabel=Strip\t509\tX=43963.80\ty=-6743.20 \nLabel=Strip\t510\tX=44314.95\ty=-6667.98 \nLabel=Strip\t511\tX=43966.09\ty=-6596.20 \nLabel=Strip\t512\tX=44317.21\ty=-6520.86 \nLabel=Strip\t513\tX=43968.33\ty=-6449.20 \nLabel=Strip\t514\tX=44319.43\ty=-6373.74 \nLabel=Strip\t515\tX=43970.52\ty=-6302.20 \nLabel=Strip\t516\tX=44321.59\ty=-6226.61 \nLabel=Strip\t517\tX=43972.66\ty=-6155.19 \nLabel=Strip\t518\tX=44323.70\ty=-6079.49 \nLabel=Strip\t519\tX=43974.75\ty=-6008.18 \nLabel=Strip\t520\tX=44325.76\ty=-5932.36 \nLabel=Strip\t521\tX=43976.79\ty=-5861.18 \nLabel=Strip\t522\tX=44327.78\ty=-5785.23 \nLabel=Strip\t523\tX=43978.77\ty=-5714.17 \nLabel=Strip\t524\tX=44329.74\ty=-5638.10 \nLabel=Strip\t525\tX=43980.71\ty=-5567.15 \nLabel=Strip\t526\tX=44331.65\ty=-5490.97 \nLabel=Strip\t527\tX=43982.60\ty=-5420.14 \nLabel=Strip\t528\tX=44333.51\ty=-5343.83 \nLabel=Strip\t529\tX=43984.43\ty=-5273.12 \nLabel=Strip\t530\tX=44335.32\ty=-5196.70 \nLabel=Strip\t531\tX=43986.22\ty=-5126.11 \nLabel=Strip\t532\tX=44337.08\ty=-5049.56 \nLabel=Strip\t533\tX=43987.95\ty=-4979.09 \nLabel=Strip\t534\tX=44338.79\ty=-4902.42 \nLabel=Strip\t535\tX=43989.64\ty=-4832.07 \nLabel=Strip\t536\tX=44340.45\ty=-4755.28 \nLabel=Strip\t537\tX=43991.27\ty=-4685.05 \nLabel=Strip\t538\tX=44342.05\ty=-4608.13 \nLabel=Strip\t539\tX=43992.85\ty=-4538.02 \nLabel=Strip\t540\tX=44343.61\ty=-4460.99 \nLabel=Strip\t541\tX=43994.39\ty=-4391.00 \nLabel=Strip\t542\tX=44345.12\ty=-4313.84 \nLabel=Strip\t543\tX=43995.87\ty=-4243.97 \nLabel=Strip\t544\tX=44346.57\ty=-4166.70 \nLabel=Strip\t545\tX=43997.30\ty=-4096.94 \nLabel=Strip\t546\tX=44347.98\ty=-4019.55 \nLabel=Strip\t547\tX=43998.68\ty=-3949.91 \nLabel=Strip\t548\tX=44349.33\ty=-3872.40 \nLabel=Strip\t549\tX=44000.02\ty=-3802.88 \nLabel=Strip\t550\tX=44350.64\ty=-3725.24 \nLabel=Strip\t551\tX=44001.30\ty=-3655.85 \nLabel=Strip\t552\tX=44351.89\ty=-3578.09 \nLabel=Strip\t553\tX=44002.53\ty=-3508.82 \nLabel=Strip\t554\tX=44353.10\ty=-3430.94 \nLabel=Strip\t555\tX=44003.71\ty=-3361.78 \nLabel=Strip\t556\tX=44354.25\ty=-3283.78 \nLabel=Strip\t
